vi "Hide Undefined Channels Write.vi"(4 "error in (no error)":errorcluster, 5 "Value":bool, 6 "Container State":T4, 7 "Display State In":T1={"Hierarchy"=[], "File/Directory Path"=path "", "Relative File Paths"=[], "Hide Undefined Channels"=FALSE, "Static File Structure"=FALSE, "Filtering"={"Filtered Groups"=[], "Group Filter Mode"=enum."Exclude", "Group Filter Regex?"=FALSE, "Filtered Channels"=[], "Channel Filter Mode"=enum."Exclude", "Channel Filter Regex?"=FALSE, "Filter Time Start"=timestamp(0 s since 1904-01-01), "Filter Time End"=timestamp(0 s since 1904-01-01), "Time Filter Mode"=enum."Include", "Time Filter Enabled"=FALSE}, "File Contents Tree"=refnum, "Properties Table"=refnum, "Loading Indicator"=refnum}) -> (0 "error out":errorcluster, 3 "Display State Out":T1={"Hierarchy"=[], "File/Directory Path"=path "", "Relative File Paths"=[], "Hide Undefined Channels"=FALSE, "Static File Structure"=FALSE, "Filtering"={"Filtered Groups"=[], "Group Filter Mode"=enum."Exclude", "Group Filter Regex?"=FALSE, "Filtered Channels"=[], "Channel Filter Mode"=enum."Exclude", "Channel Filter Regex?"=FALSE, "Filter Time Start"=timestamp(0 s since 1904-01-01), "Filter Time End"=timestamp(0 s since 1904-01-01), "Time Filter Mode"=enum."Include", "Time Filter Enabled"=FALSE}, "File Contents Tree"=refnum, "Properties Table"=refnum, "Loading Indicator"=refnum})   [LabVIEW 2017, in "XTree.xctl"]
doc: "Hide channels which are missing any of the properties specified in the hierarchy"
uses:
  <vilib>/addons/_NIFileIO/XTree/XTree.xctl
  <vilib>/_xctls/Container State.ctl
  <vilib>/addons/_NIFileIO/XTree/State.ctl
  <vilib>/addons/_NIFileIO/XTree/Controls/Filter Settings.ctl
  <vilib>/addons/_NIFileIO/XTree/Controls/Filter Mode.ctl
  <vilib>/_xctls/XControlSupport.lvlib
panel:
  # "Replace the Value Control below with a Control of desired type.\nDo not remove this Control or the others from the connector pane.\nDo not change the connector pane pattern.\nThe Value control should always be the third terminal from top on the input side in the connector pane."
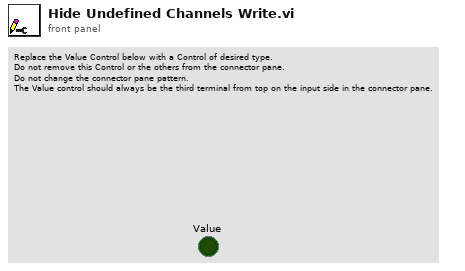
[diagram p1: front panel]
types:
  T1 = typedef "XTree.xctl/State.ctl" = cluster{"Hierarchy":string[], "File/Directory Path":path, "Relative File Paths":string[], "Hide Undefined Channels":bool, "Static File Structure":bool, "Filtering":T2, "File Contents Tree":refnum<vi>, "Properties Table":refnum<vi>, "Loading Indicator":refnum<vi>}
  T2 = typedef "XTree.xctl/Filter Settings.ctl" = cluster{"Filtered Groups":string[], "Group Filter Mode":T3, "Group Filter Regex?":bool, "Filtered Channels":string[], "Channel Filter Mode":T3, "Channel Filter Regex?":bool, "Filter Time Start":timestamp, "Filter Time End":timestamp, "Time Filter Mode":T3, "Time Filter Enabled":bool}
  T3 = typedef "XTree.xctl/Filter Mode.ctl" = enum16{"Exclude", "Include"}
  T4 = typedef "XControlSupport.lvlib/Container State.ctl" = cluster{"Indicator?":bool, "Run Mode?":bool, " Refnum":refnum<vi>}
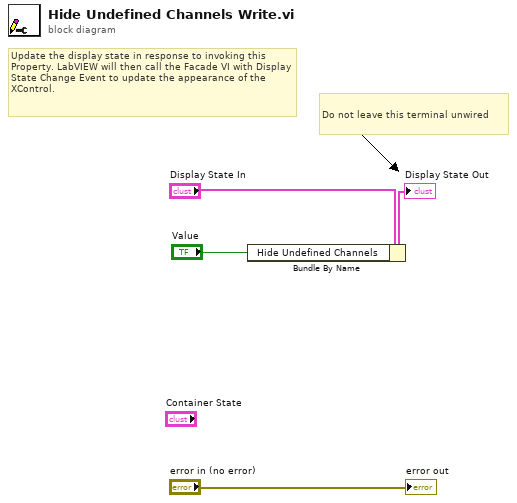
[diagram p0: block diagram]
diagram:
  # "Do not leave this terminal unwired"
  # "Update the display state in response to invoking this Property. LabVIEW will then call the Facade VI with Display State Change Event to update the appearance of the XControl."
  n1 = Bundle By Name(cluster="Display State In", "Hide Undefined Channels"="Value") -> (→"Display State Out":T1)
  "error out" <- "error in (no error)"
